vi "Codec_CMD_24.vi"(8 "error in (no error)":errorcluster, 10 "AskCMD24":T1={"STATION"="F/T-B", "RACK"="101", "DUT"="1", "SN"="AP32023099", "MAC_BMC"="2D;MAC1;AC81B504A499", "MAC_SWITCH"="AC81B502F1B4", "MAC_SCM"="AC81B504A474"}, 11 "SecureMqttCodec in":refnum<class "SecureMqttCodec.lvclass">) -> (0 "error out":errorcluster, 2 "<JSON>":string="{\r  \"CMD\": 24,\r  \"CONTENT\": [\r    {\r      \"DUT\": \"1\",\r      \"MAC_BMC\": \"2D;MAC1;AC81B504A499\",\r      \"MAC_SCM\": \"AC81B504A474\",\r      \"MAC_SWITCH\": \"AC81B502F1B4\",\r      \"RACK\": \"101\",\r      \"SN\": \"AP32023099\",\r      \"STATION\": \"F/T-B\"\r    }\r  ],\r  \"ERRCODE\": \"\",\r  \"ERRMSG\": \"\",\r  \"FROM\": \"845CF3525B43\",\r  \"ID\": \"8B8F30BF-9F76-4CF5-AA91-F98ABDE8E26A\",\r  \"STATUS\": \"\",\r  \"TIMESTAMP\": 1759592287,\r  \"TO\": \"\"\r}", 3 "SecureMqttCodec out":refnum<class "SecureMqttCodec.lvclass">)   [LabVIEW 2020, in "SecureMqttCodec.lvclass"]
uses:
  SecureMqttCodec.lvclass
  <vilib>/addons/JSON API/JSON Object/JSON Object.lvclass
  <vilib>/addons/JSON API/JSON Scalar/JSON Scalar.lvclass
  C:/Program Files/National Instruments/LabVIEW 2020/vi.lib/addons/JSON API/JSON Value/JSON Value.lvclass
  TestMQTT/Ctrl/ReplyCMD24.ctl
  SecureMqttCodec.lvclass/SecureMqttCodec.ctl
  <vilib>/addons/JSON API/JSON Value/Set from JSON string.vi
  <vilib>/addons/JSON API/JSON Array/JSON Array.lvclass
  <vilib>/addons/JSON API/JSON Scalar/Set U32.vi
  <vilib>/addons/JSON API/JSON Array/Set JSON Array.vi
  <vilib>/addons/JSON API/JSON Value/Get as JSON string (pretty).vi
  <vilib>/addons/JSON API/JSON Value/JSON Value.lvclass
  <vilib>/addons/JSON API/Get Polymorphic/JSON GetSet.lvlib
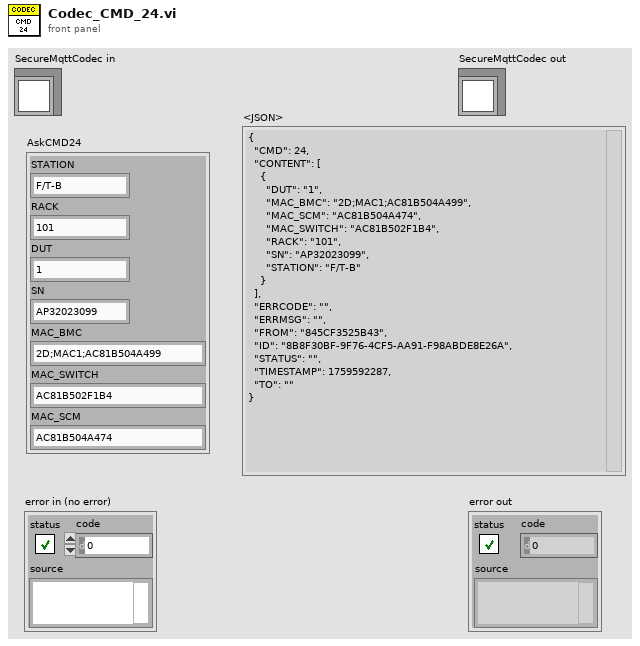
[diagram p1: front panel]
types:
  T1 = typedef "ReplyCMD24.ctl" = cluster{"STATION":string, "RACK":string, "DUT":string, "SN":string, "MAC_BMC":string, "MAC_SWITCH":string, "MAC_SCM":string}
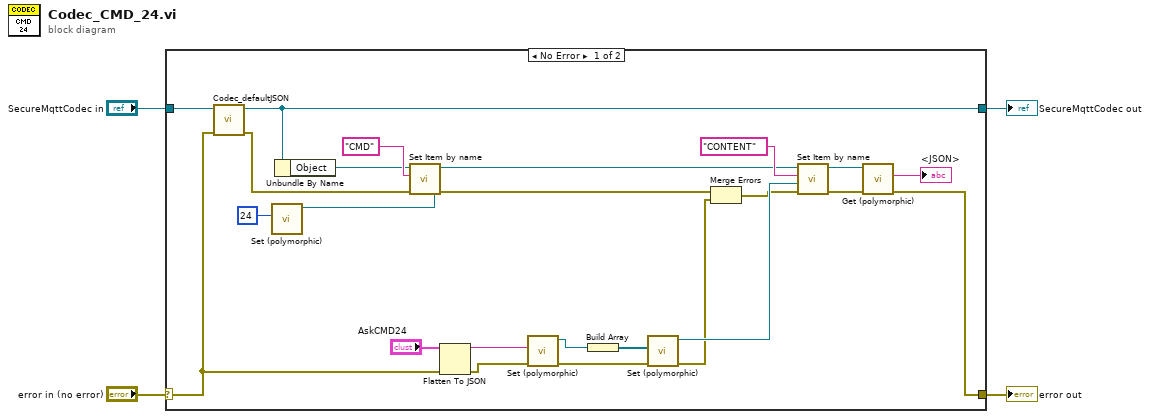
[diagram p0: block diagram]
diagram:
  n1 = case shown="No Error" "error in (no error)" {
    selector: "error in (no error)" -> [w12 w30]
    tunnel: [w25 w30] -> w3
    tunnel: [w18 w29] -> w1
    tunnel: "SecureMqttCodec in" -> [w28 w29]
    frame No Error {
      n2 = call "Codec_defaultJSON.vi"("error in (no error)"=w12, "SecureMqttCodec in"=w28) -> ("error out"=w17:errorcluster, "SecureMqttCodec out"=w18:refnum<class "SecureMqttCodec.lvclass">)  [unwired: 8 in]
      n3 = call-poly <vilib>:"Set (polymorphic).vi"("Numeric"=u32 24) -> ("JSON Scalar out"=w26:refnum<class "JSON Scalar.lvclass">)  [unwired: 9 in, 1 out]
      n4 = Unbundle By Name(w18) -> ("Object"=w6:refnum<class "JSON Value.lvclass">)
      n5 = call-dynamic "Set Item by name.vi"("error in (no error)"=w17, "Value"=w26, "name"="CMD", "JSON Value In"=w6) -> ("error out"=w22:errorcluster, "JSON Value Out"=w7:refnum<class "JSON Value.lvclass">)  [unwired: 5 in, 1 out]
      n6 = Flatten To JSON(anything="AskCMD24", error in (no error)=w12) -> (JSON string=w14:string, 11:w13:errorcluster)  [unwired: 1 in]
      n7 = call-poly <vilib>:"Set (polymorphic).vi"("error in (no error)"=w13, "JSON stream"=w14) -> ("error out"=w11:errorcluster, "JSON Value out"=w5:refnum<class "JSON Value.lvclass">)  [unwired: 7 in, 1 out]
      n8 = Build Array(w5) -> (w15:refnum<class "JSON Value.lvclass">[])
      n9 = call-poly <vilib>:"Set (polymorphic).vi"("error in (no error)"=w11, "Array"=w15) -> ("error out"=w9:errorcluster, "JSON Array out"=w20:refnum<class "JSON Array.lvclass">)  [unwired: 8 in]
      n10 = Merge Errors(w22, w9) -> (w10:errorcluster)
      n11 = call-dynamic "Set Item by name.vi"("error in (no error)"=w10, "Value"=w20, "name"="CONTENT", "JSON Value In"=w7) -> ("error out"=w21:errorcluster, "JSON Value Out"=w23:refnum<class "JSON Value.lvclass">)  [unwired: 5 in, 1 out]
      n12 = call-poly <vilib>:"Get (polymorphic).vi"("error in (no error)"=w21, "JSON Value in"=w23) -> ("error out"=w25:errorcluster, "<JSON>"=→"<JSON>":string)  [unwired: 8 in]
    }
    frame Error {
    }
  }
  "error out" <- w3
  "SecureMqttCodec out" <- w1
